vi "Stock Table - Animate.vi"(8 "error in":errorcluster, 11 "Table Reference":refnum<vi>) -> (0 "error out":errorcluster)   [LabVIEW 2011]
doc: "'Animate' the table by changing the background colour of selected table cells.\nGreen if the value is positive and red otherwise.\n\nInputs:\n Table Reference: Reference to a table \n Error in: Describes error conditions that occur before this node runs. This input provides standard error in functionality.\n\nOutputs:\n Error out: Contains error information. This output provides standard error out functionality."
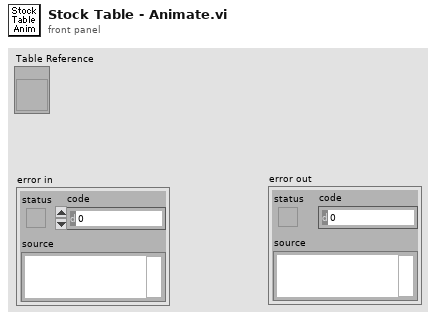
[diagram p1: front panel]
types:
  T1 = enum16{"Symbol", "Name", "Price", "Change", "Change %", "Volume"}
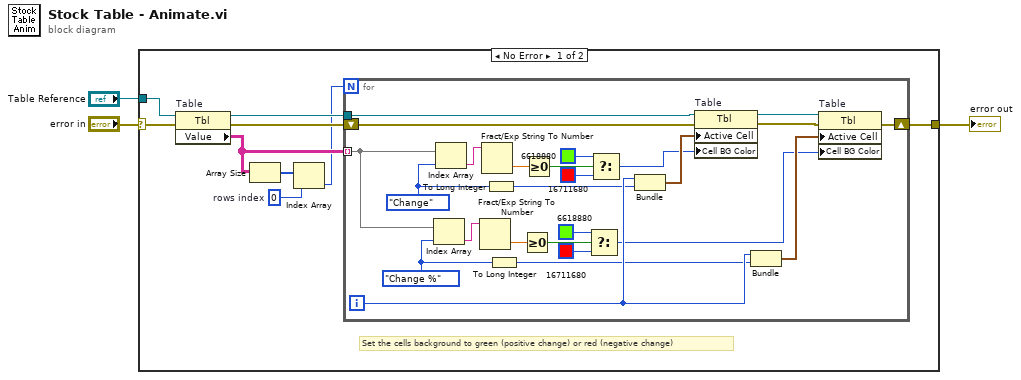
[diagram p0: block diagram]
diagram:
  n1 = case shown="No Error" "error in" {
    selector: "error in" -> [w4 w38]
    tunnel: "Table Reference" -> [w5 _]
    tunnel: [w11 w38] -> w3
    frame No Error {
      w7 = 0  # rows index
      # "Set the cells background to green (positive change) or red (negative change)"
      n2 = property on="Table" class="Tbl"(reference=w5, error in=w4) -> (reference out=w10:refnum<vi>, error out=w12:errorcluster, "Value"=w9:string[][])
      n3 = Array Size(array=w9) -> (size(s)=w8:i32[])
      n4 = Index Array(array=w8, index=w7) -> (element=w6:i32)
      n5 = for {
        N: w6 -> [_]
        shift-right: [w18] -> w11
        shift-left: w12 -> [w19]
        tunnel: w9 -> [w27] mode=indexing
        tunnel: w10 -> [w14]
        i -> [w24]
        w26 = T1."Change %"
        w25 = T1."Change"
        n6 = Index Array(array=w27, index=w26) -> (element=w32:string)
        n7 = Index Array(array=w27, index=w25) -> (element=w37:string)
        n8 = Fract/Exp String To Number(string=w32) -> (number=w28:dbl)  [unwired: 3 in, 1 out]
        n9 = Fract/Exp String To Number(string=w37) -> (number=w33:dbl)  [unwired: 3 in, 1 out]
        n10 = To Long Integer(number=w25) -> (32bit integer=w23:i32)
        n11 = To Long Integer(number=w26) -> (32bit integer=w22:i32)
        n12 = Greater Or Equal To 0?(x=w28) -> (x >= 0?=w31:bool)
        n13 = Greater Or Equal To 0?(x=w33) -> (x >= 0?=w36:bool)
        n14 = Select(t=u32 6618880, s=w31, f=u32 16711680) -> (s? t:f=w15:u32)
        n15 = Select(t=u32 6618880, s=w36, f=u32 16711680) -> (s? t:f=w20:u32)
        n16 = Bundle(w24, w23) -> (w21:cluster{i32, i32})  [unwired: 1 in]
        n17 = property on="Table" class="Tbl"(reference=w14, error in=w19, "Active Cell"=w21, "Cell BG Color"=w20) -> (reference out=w13:refnum<vi>, error out=w17:errorcluster)
        n18 = Bundle(w24, w22) -> (w16:cluster{i32, i32})  [unwired: 1 in]
        n19 = property on="Table" class="Tbl"(reference=w13, error in=w17, "Active Cell"=w16, "Cell BG Color"=w15) -> (error out=w18:errorcluster)  [unwired: 1 out]
      }
    }
    frame Error {
    }
  }
  "error out" <- w3
